vi "IsNoReceiveError.vi"(11 "Packet":T1) -> (3 "IsNotReceived?":bool)   [LabVIEW 2009]
uses:
  Packet.ctl
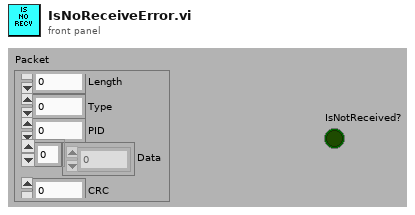
[diagram p1: front panel]
types:
  T1 = typedef "Packet.ctl" = cluster{"Length":u8, "Type":u8, "PID":u8, "Data":u8[], "CRC":u8}
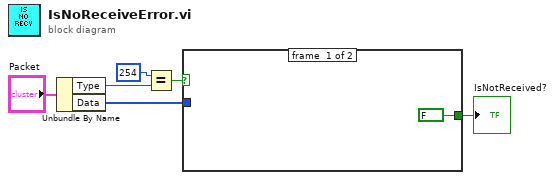
[diagram p0: block diagram]
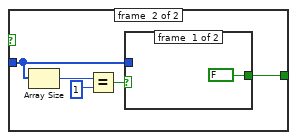
[diagram p2: hidden frame]
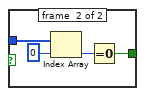
[diagram p3: hidden frame]
diagram:
  n1 = Unbundle By Name("Packet") -> ("Type"=w5:u8, "Data"=w1:u8[])
  n2 = Equal?(x=u8 254, y=w5) -> (x = y?=w3:bool)
  n3 = case shown="True" w3 {
    tunnel: [FALSE ("IsNotReceived?") w9] -> w2
    tunnel: w1 -> [_ w8]
    frame #0 {
    }
    frame #1 {
      n4 = Array Size(array=w8) -> (size(s)=w12:i32)
      n5 = Equal?(x=w12, y=1) -> (x = y?=w10:bool)
      n6 = case shown="True" w10 {
        tunnel: [FALSE ("IsNotReceived?") w14] -> w9
        tunnel: w8 -> [_ w17]
        frame #0 {
        }
        frame #1 {
          n7 = Index Array(array=w17, index=0) -> (element=w15:u8)
          n8 = Equal To 0?(x=w15) -> (x = 0?=w14:bool)
        }
      }
    }
  }
  "IsNotReceived?" <- w2
